vi "Robot Global Data.vi"() -> ()   [LabVIEW 2011]
doc: "This global VI can contain as many global variables as you need. Place a control on the panel, give it a good name. To read or write to it from a VI, drag the icon to the diagram of that VI. You can also drag from the project. Click on the node to change which global you access. You shouldn't have multiple locations writing to a global or it will cause a race-condition."
panel:
  out "RPM":dbl
  out "RPM -250":bool
  out "RPM +250":bool
  out "Bad Shot":bool
  out "Max":bool=TRUE
  out "Poop":bool=TRUE
  out "Encoder Right Rate":dbl
  out "Encoder Left Rate":dbl
  out "Turret Button 5":bool
  out "Turret Button 6":bool
  out "Shoot All":bool
  in  "SpinerOptions":enum16{"Full", "16", "14", "12", "Poop"}(ring)=enum."14"
  in  "BallActionNew":T1(ring)
  out "Encoder3 Rate":dbl
  out "Motor Reverse":bool
  in  "EncoderRight":dbl
  in  "EncoderLeft":dbl
  out "Tipper Buttons":i32
  out "Shoot":bool
  out "Turret Joystick X-Axis":dbl
  out "Load":bool
  out "14 Foot":bool=TRUE
  out "12 Foot":bool=TRUE
  out "16 Foot":bool=TRUE
  out "Tacometer":dbl
  out "Encoder4 Rate":dbl
  in  "LED toggle rate (ms)":u32=100
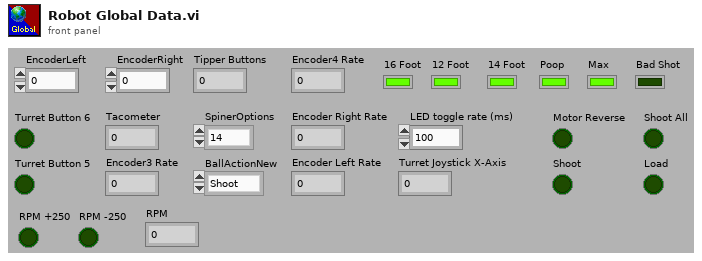
[diagram p1: front panel]
types:
  T1 = enum16{"Shoot", "Load", "Arm", "Nothing", "Reverse", "ShootAll"}
diagram:
